vi "LT_get_315_SN.vi"(8 "error in":errorcluster, 10 "dev_param_in":T1={"Length of data block (14)"=14, "Converter address (0)"=0, "Converter type\n(180: Turbovac 350/450 i)"=180, "PZD1 STW, ZSW (0)"=0, "PZD2 HSW, HIW (0)"=0} {"Converter type\n(180: Turbovac 350/450 i)" items=["Turbovac 350/450 i"=180, "Turbovac 350/450 i with optional interface"=181, "Turbovac 350/450 iX"=182, "Turbovac  90/250 i"=190, "Turbovac  90/250 with optional interface"=191, "Turbovac  90/250 iX"=192, "Turbovac  850/950 i"=195, "Turbovac  850/950 i with optional interface"=196, "Turbovac  850/950 iX"=197, "Turbovac 1350/1450 i"=185, "Turbovac 1350/1450 i with optional interface"=186, "Turbovac 1350/1450 iX"=187]; "Length of data block (14)" items=["14"=14, "22"=22]}, 11 "VISA in":refnum<visa-resource-name>="COM43") -> (0 "error out":errorcluster, 2 "dev_param_out":T3={"Length of data block"=14, "Converter address"=0, "Converter type"=180, "PZD1"=0, "PZD2"=0} {"Converter type" items=["Turbovac 350/450 i"=180, "Turbovac 350/450 i with optional interface"=181, "Turbovac 350/450 iX"=182, "Turbovac  90/250 i"=190, "Turbovac  90/250 with optional interface"=191, "Turbovac  90/250 iX"=192, "Turbovac  850/950 i"=195, "Turbovac  850/950 i with optional interface"=196, "Turbovac  850/950 iX"=197, "Turbovac 1350/1450 i"=185, "Turbovac 1350/1450 i with optional interface"=186, "Turbovac 1350/1450 iX"=187]; "Length of data block" items=["14"=14, "22"=22]}, 3 "VISA out":refnum<visa-resource-name>, 4 "SN_converter":string)   [LabVIEW 2019]
doc: "Example VI to demonstrate the use of the Oerlikon Leybold TMP driver."
uses:
  <instrlib>/Leybold TURBOVAC/Public/Ctl/Device Parameters Indicator.ctl
  <instrlib>/Leybold TURBOVAC/Public/Ctl/Converter Type Indicator.ctl
  <instrlib>/Leybold TURBOVAC/Public/Ctl/Device Parameters Control.ctl
  <instrlib>/Leybold TURBOVAC/Public/Ctl/Converter Type Control.ctl
  <instrlib>/Leybold TURBOVAC/Leybold TURBOVAC.lvlib
panel:
  out "chars":string[](array[string])
  out "values":i8[](array[numeric])
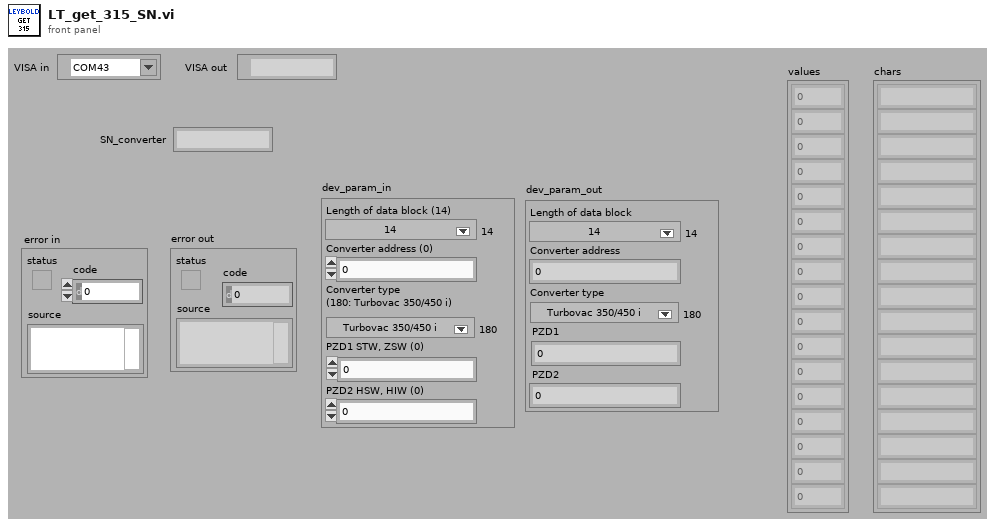
[diagram p1: front panel]
types:
  T1 = typedef "Leybold TURBOVAC.lvlib/Device Parameters Control.ctl" = cluster{"Length of data block (14)":u8, "Converter address (0)":u8, "Converter type\n(180: Turbovac 350/450 i)":T2, "PZD1 STW, ZSW (0)":u16, "PZD2 HSW, HIW (0)":u16}
  T2 = typedef "Leybold TURBOVAC.lvlib/Converter Type Control.ctl" = u16
  T3 = typedef "Leybold TURBOVAC.lvlib/Device Parameters Indicator.ctl" = cluster{"Length of data block":u8, "Converter address":u8, "Converter type":T4, "PZD1":u16, "PZD2":u16}
  T4 = typedef "Leybold TURBOVAC.lvlib/Converter Type Indicator.ctl" = u16
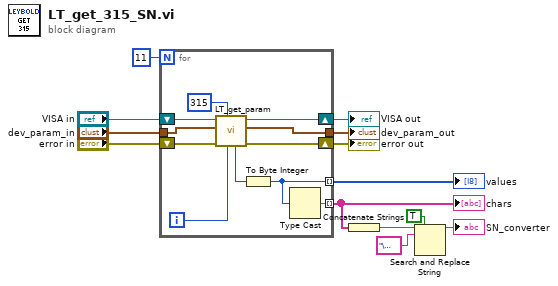
[diagram p0: block diagram]
diagram:
  n1 = for {
    N: 11 -> [_]
    tunnel: "dev_param_in" -> [w20]
    tunnel: [w19] -> w9
    shift-right: [w22] -> w12
    shift-left: "VISA in" -> [w23]
    shift-right: [w18] -> w8
    shift-left: "error in" -> [w21]
    tunnel: [w14] -> w6 mode=indexing
    tunnel: [w17] -> w5 mode=indexing
    i -> [w16]
    n2 = call "LT_get_param.vi"("param_index"=w16, "param_number"=u16 315, "error in"=w21, "dev_param_in"=w20, "VISA in"=w23) -> ("error out"=w18:errorcluster, "dev_param_out"=w19:T3, "VISA out"=w22:refnum<visa-resource-name>, "PWE"=w15:i32)  [unwired: 3 in]
    n3 = To Byte Integer(number=w15) -> (8bit integer=w14:i8)
    n4 = Type Cast(x=w14) -> (*(type *) &x=w17:string)  [unwired: 1 in]
  }
  "VISA out" <- w12
  "dev_param_out" <- w9
  "error out" <- w8
  "values" <- w6
  "chars" <- w5
  n5 = Concatenate Strings(w5) -> (w4:string)
  n6 = Search and Replace String(replace all?=TRUE ("replace all? (F)"), input string=w4, search string="\u0000") -> (result string=→"SN_converter":string)  [unwired: 5 in, 3 out]
